vi "Lab Panel V4.88.vi"() -> ()   [LabVIEW 2013] (continued)
                            n2188 = Build Array(w4041) -> (w4037:dbl[])
                            n2189 = Build Array(w4039) -> (w4036:dbl[])
                            n2190 = Build Array(w4044) -> (w4031:dbl[])
                            n2191 = Build Array("AMPS ON", "AMPS OFF", "VOLTS", "PF", "TEMP Live", "TEMP Neut", "CYCLE") -> (w4014:string[])
                            n2192 = Bundle By Name("Y"=w4037, "t0"=w4030) -> (w4029:waveform(dbl))  [unwired: 1 in]
                            n2193 = Bundle By Name("Y"=w4036, "t0"=w4030) -> (w4028:waveform(dbl))  [unwired: 1 in]
                            n2194 = Bundle By Name("Y"=w4035, "t0"=w4030) -> (w4027:waveform(dbl))  [unwired: 1 in]
                            n2195 = Bundle By Name("Y"=w4034, "t0"=w4030) -> (w4026:waveform(dbl))  [unwired: 1 in]
                            n2196 = Bundle By Name("Y"=w4033, "t0"=w4030) -> (w4025:waveform(dbl))  [unwired: 1 in]
                            n2197 = Bundle By Name("Y"=w4032, "t0"=w4030) -> (w4024:waveform(dbl))  [unwired: 1 in]
                            n2198 = Bundle By Name("Y"=w4031, "t0"=w4030) -> (w4023:waveform(dbl))  [unwired: 1 in]
                            n2199 = Build Array(w4029, w4028, w4027, w4026, w4025, w4024, w4023) -> (w4022:waveform(dbl)[])
                            n2200 = TDMS Write(0:w4043, 5:"TEST VALUES", 7:w4014, 9:w4022) -> (4:w4013:refnum<k34>, 6:w4012:string, 15:w4011:errorcluster)  [unwired: 2 in, 1 out]
                            n2201 = TDMS Write(0:w4013, 5:w4012, 7:"TIME", 9:w4009, 11:w4011) -> (15:w4008:errorcluster)  [unwired: 1 in, 3 out]
                            n2202 = local write "data file error"(w4008) -> ()
                          }
                        }
                      }
                    }
                  }
                }
              }
              frame #4 {
                n2203 = case shown="True" w4047 {
                  tunnel: w4051 -> [_ w4056]
                  tunnel: w4050 -> [_ w4055]
                  tunnel: w4049 -> [_ w4053]
                  tunnel: w4048 -> [_ w4052]
                  frame False {
                  }
                  frame True {
                    n2204 = local read "DISP LAB03-1"() -> (w4057:T4)
                    n2205 = local read "SIG LAB03-1"() -> (w4058:T2)
                    n2206 = local read "ON L03-1"() -> (w4054:cluster{"amps":dbl, "volts":dbl, "pf":dbl})
                    n2207 = Unbundle(w4058) -> ("AMPS"=w4064:dbl, "VOLTS"=w4062:dbl, "PF"=w4061:dbl, "Tmp Live"=w4060:dbl, "Tmp Neut"=w4063:dbl)
                    n2208 = Unbundle(w4057) -> ("CYCLE"=w4059:dbl)  [unwired: 2 out]
                    n2209 = stacked-sequence {
                      tunnel: w4064 -> [w4068 w4087]
                      tunnel: w4063 -> [_ w4086]
                      tunnel: w4062 -> [w4067 w4085]
                      tunnel: w4061 -> [w4066 w4084]
                      tunnel: w4060 -> [_ w4083]
                      tunnel: w4059 -> [_ w4082]
                      tunnel: w4056 -> [_ w4081]
                      tunnel: w4055 -> [w4069 _]
                      tunnel: w4054 -> [w4065 w4079]
                      tunnel: w4053 -> [_ w4080]
                      tunnel: w4052 -> [_ w4075]
                      frame #0 {
                        n2210 = case shown="True" w4069 {
                          tunnel: w4068 -> [_ w4074]
                          tunnel: w4067 -> [_ w4073]
                          tunnel: w4066 -> [_ w4072]
                          tunnel: w4065 -> [_ w4070]
                          frame False {
                          }
                          frame True {
                            n2211 = Bundle(cluster=w4070, "amps"=w4074, "volts"=w4073, "pf"=w4072) -> (w4071:cluster{"amps":dbl, "volts":dbl, "pf":dbl})
                            n2212 = local write "ON L03-1"(w4071) -> ()
                          }
                        }
                      }
                      frame #1 {
                        n2213 = Unbundle(w4079) -> ("amps"=w4078:dbl, "volts"=w4077:dbl, "pf"=w4076:dbl)
                        n2214 = case shown="True" w4080 {
                          tunnel: w4087 -> [_ w4119]
                          tunnel: w4086 -> [_ w4126]
                          tunnel: w4085 -> [_ _]
                          tunnel: w4084 -> [_ _]
                          tunnel: w4083 -> [_ w4125]
                          tunnel: w4082 -> [_ w4124]
                          tunnel: w4081 -> [_ w4089]
                          tunnel: w4078 -> [_ w4121]
                          tunnel: w4077 -> [_ w4120]
                          tunnel: w4076 -> [_ w4118]
                          tunnel: w4075 -> [_ w4110]
                          frame False {
                          }
                          frame True {
                            n2215 = local read "TDMS LAB03-1"() -> (w4123:refnum<k34>)
                            n2216 = Build Array(w4120) -> (w4115:dbl[])
                            n2217 = Build Array(w4118) -> (w4114:dbl[])
                            n2218 = Build Array(w4125) -> (w4113:dbl[])
                            n2219 = Build Array(w4126) -> (w4112:dbl[])
                            n2220 = Build Array(w4121) -> (w4117:dbl[])
                            n2221 = Build Array(w4119) -> (w4116:dbl[])
                            n2222 = Build Array(w4124) -> (w4111:dbl[])
                            n2223 = Build Array("AMPS ON", "AMPS OFF", "VOLTS", "PF", "TEMP Live", "TEMP Neut", "CYCLE") -> (w4094:string[])
                            n2224 = Bundle By Name("Y"=w4117, "t0"=w4110) -> (w4109:waveform(dbl))  [unwired: 1 in]
                            n2225 = Bundle By Name("Y"=w4116, "t0"=w4110) -> (w4108:waveform(dbl))  [unwired: 1 in]
                            n2226 = Bundle By Name("Y"=w4115, "t0"=w4110) -> (w4107:waveform(dbl))  [unwired: 1 in]
                            n2227 = Bundle By Name("Y"=w4114, "t0"=w4110) -> (w4106:waveform(dbl))  [unwired: 1 in]
                            n2228 = Bundle By Name("Y"=w4113, "t0"=w4110) -> (w4105:waveform(dbl))  [unwired: 1 in]
                            n2229 = Bundle By Name("Y"=w4112, "t0"=w4110) -> (w4104:waveform(dbl))  [unwired: 1 in]
                            n2230 = Bundle By Name("Y"=w4111, "t0"=w4110) -> (w4103:waveform(dbl))  [unwired: 1 in]
                            n2231 = Build Array(w4109, w4108, w4107, w4106, w4105, w4104, w4103) -> (w4102:waveform(dbl)[])
                            n2232 = TDMS Write(0:w4123, 5:"TEST VALUES", 7:w4094, 9:w4102) -> (4:w4093:refnum<k34>, 6:w4092:string, 15:w4091:errorcluster)  [unwired: 2 in, 1 out]
                            n2233 = TDMS Write(0:w4093, 5:w4092, 7:"TIME", 9:w4089, 11:w4091) -> (15:w4088:errorcluster)  [unwired: 1 in, 3 out]
                            n2234 = local write "data file error"(w4088) -> ()
                          }
                        }
                      }
                    }
                  }
                }
              }
              frame #5 {
                n2235 = case shown="True" w4127 {
                  tunnel: w4131 -> [_ w4136]
                  tunnel: w4130 -> [_ w4135]
                  tunnel: w4129 -> [_ w4133]
                  tunnel: w4128 -> [_ w4132]
                  frame False {
                  }
                  frame True {
                    n2236 = local read "DISP LAB03-2"() -> (w4137:T4)
                    n2237 = local read "SIG LAB03-2"() -> (w4138:T2)
                    n2238 = local read "ON L03-2"() -> (w4134:cluster{"amps":dbl, "volts":dbl, "pf":dbl})
                    n2239 = Unbundle(w4138) -> ("AMPS"=w4144:dbl, "VOLTS"=w4142:dbl, "PF"=w4141:dbl, "Tmp Live"=w4140:dbl, "Tmp Neut"=w4143:dbl)
                    n2240 = Unbundle(w4137) -> ("CYCLE"=w4139:dbl)  [unwired: 2 out]
                    n2241 = stacked-sequence {
                      tunnel: w4144 -> [w4148 w4167]
                      tunnel: w4143 -> [_ w4166]
                      tunnel: w4142 -> [w4147 w4165]
                      tunnel: w4141 -> [w4146 w4164]
                      tunnel: w4140 -> [_ w4163]
                      tunnel: w4139 -> [_ w4162]
                      tunnel: w4136 -> [_ w4161]
                      tunnel: w4135 -> [w4149 _]
                      tunnel: w4134 -> [w4145 w4159]
                      tunnel: w4133 -> [_ w4160]
                      tunnel: w4132 -> [_ w4155]
                      frame #0 {
                        n2242 = case shown="True" w4149 {
                          tunnel: w4148 -> [_ w4154]
                          tunnel: w4147 -> [_ w4153]
                          tunnel: w4146 -> [_ w4152]
                          tunnel: w4145 -> [_ w4150]
                          frame False {
                          }
                          frame True {
                            n2243 = Bundle(cluster=w4150, "amps"=w4154, "volts"=w4153, "pf"=w4152) -> (w4151:cluster{"amps":dbl, "volts":dbl, "pf":dbl})
                            n2244 = local write "ON L03-2"(w4151) -> ()
                          }
                        }
                      }
                      frame #1 {
                        n2245 = Unbundle(w4159) -> ("amps"=w4158:dbl, "volts"=w4157:dbl, "pf"=w4156:dbl)
                        n2246 = case shown="True" w4160 {
                          tunnel: w4167 -> [_ w4199]
                          tunnel: w4166 -> [_ w4206]
                          tunnel: w4165 -> [_ _]
                          tunnel: w4164 -> [_ _]
                          tunnel: w4163 -> [_ w4205]
                          tunnel: w4162 -> [_ w4204]
                          tunnel: w4161 -> [_ w4169]
                          tunnel: w4158 -> [_ w4201]
                          tunnel: w4157 -> [_ w4200]
                          tunnel: w4156 -> [_ w4198]
                          tunnel: w4155 -> [_ w4190]
                          frame False {
                          }
                          frame True {
                            n2247 = local read "TDMS LAB03-2"() -> (w4203:refnum<k34>)
                            n2248 = Build Array(w4200) -> (w4195:dbl[])
                            n2249 = Build Array(w4198) -> (w4194:dbl[])
                            n2250 = Build Array(w4205) -> (w4193:dbl[])
                            n2251 = Build Array(w4206) -> (w4192:dbl[])
                            n2252 = Build Array(w4201) -> (w4197:dbl[])
                            n2253 = Build Array(w4199) -> (w4196:dbl[])
                            n2254 = Build Array(w4204) -> (w4191:dbl[])
                            n2255 = Build Array("AMPS ON", "AMPS OFF", "VOLTS", "PF", "TEMP Live", "TEMP Neut", "CYCLE") -> (w4174:string[])
                            n2256 = Bundle By Name("Y"=w4197, "t0"=w4190) -> (w4189:waveform(dbl))  [unwired: 1 in]
                            n2257 = Bundle By Name("Y"=w4196, "t0"=w4190) -> (w4188:waveform(dbl))  [unwired: 1 in]
                            n2258 = Bundle By Name("Y"=w4195, "t0"=w4190) -> (w4187:waveform(dbl))  [unwired: 1 in]
                            n2259 = Bundle By Name("Y"=w4194, "t0"=w4190) -> (w4186:waveform(dbl))  [unwired: 1 in]
                            n2260 = Bundle By Name("Y"=w4193, "t0"=w4190) -> (w4185:waveform(dbl))  [unwired: 1 in]
                            n2261 = Bundle By Name("Y"=w4192, "t0"=w4190) -> (w4184:waveform(dbl))  [unwired: 1 in]
                            n2262 = Bundle By Name("Y"=w4191, "t0"=w4190) -> (w4183:waveform(dbl))  [unwired: 1 in]
                            n2263 = Build Array(w4189, w4188, w4187, w4186, w4185, w4184, w4183) -> (w4182:waveform(dbl)[])
                            n2264 = TDMS Write(0:w4203, 5:"TEST VALUES", 7:w4174, 9:w4182) -> (4:w4173:refnum<k34>, 6:w4172:string, 15:w4171:errorcluster)  [unwired: 2 in, 1 out]
                            n2265 = TDMS Write(0:w4173, 5:w4172, 7:"TIME", 9:w4169, 11:w4171) -> (15:w4168:errorcluster)  [unwired: 1 in, 3 out]
                            n2266 = local write "data file error"(w4168) -> ()
                          }
                        }
                      }
                    }
                  }
                }
              }
              frame #6 {
                n2267 = case shown="True" w4207 {
                  tunnel: w4211 -> [_ w4216]
                  tunnel: w4210 -> [_ w4215]
                  tunnel: w4209 -> [_ w4213]
                  tunnel: w4208 -> [_ w4212]
                  frame False {
                  }
                  frame True {
                    n2268 = local read "DISP LAB04-1"() -> (w4217:T4)
                    n2269 = local read "SIG LAB04-1"() -> (w4218:T2)
                    n2270 = local read "ON L04-1"() -> (w4214:cluster{"amps":dbl, "volts":dbl, "pf":dbl})
                    n2271 = Unbundle(w4218) -> ("AMPS"=w4224:dbl, "VOLTS"=w4222:dbl, "PF"=w4221:dbl, "Tmp Live"=w4220:dbl, "Tmp Neut"=w4223:dbl)
                    n2272 = Unbundle(w4217) -> ("CYCLE"=w4219:dbl)  [unwired: 2 out]
                    n2273 = stacked-sequence {
                      tunnel: w4224 -> [w4228 w4247]
                      tunnel: w4223 -> [_ w4246]
                      tunnel: w4222 -> [w4227 w4245]
                      tunnel: w4221 -> [w4226 w4244]
                      tunnel: w4220 -> [_ w4243]
                      tunnel: w4219 -> [_ w4242]
                      tunnel: w4216 -> [_ w4241]
                      tunnel: w4215 -> [w4229 _]
                      tunnel: w4214 -> [w4225 w4239]
                      tunnel: w4213 -> [_ w4240]
                      tunnel: w4212 -> [_ w4235]
                      frame #0 {
                        n2274 = case shown="True" w4229 {
                          tunnel: w4228 -> [_ w4234]
                          tunnel: w4227 -> [_ w4233]
                          tunnel: w4226 -> [_ w4232]
                          tunnel: w4225 -> [_ w4230]
                          frame False {
                          }
                          frame True {
                            n2275 = Bundle(cluster=w4230, "amps"=w4234, "volts"=w4233, "pf"=w4232) -> (w4231:cluster{"amps":dbl, "volts":dbl, "pf":dbl})
                            n2276 = local write "ON L04-1"(w4231) -> ()
                          }
                        }
                      }
                      frame #1 {
                        n2277 = Unbundle(w4239) -> ("amps"=w4238:dbl, "volts"=w4237:dbl, "pf"=w4236:dbl)
                        n2278 = case shown="True" w4240 {
                          tunnel: w4247 -> [_ w4279]
                          tunnel: w4246 -> [_ w4286]
                          tunnel: w4245 -> [_ _]
                          tunnel: w4244 -> [_ _]
                          tunnel: w4243 -> [_ w4285]
                          tunnel: w4242 -> [_ w4284]
                          tunnel: w4241 -> [_ w4249]
                          tunnel: w4238 -> [_ w4281]
                          tunnel: w4237 -> [_ w4280]
                          tunnel: w4236 -> [_ w4278]
                          tunnel: w4235 -> [_ w4270]
                          frame False {
                          }
                          frame True {
                            n2279 = local read "TDMS LAB04-1"() -> (w4283:refnum<k34>)
                            n2280 = Build Array(w4280) -> (w4275:dbl[])
                            n2281 = Build Array(w4278) -> (w4274:dbl[])
                            n2282 = Build Array(w4285) -> (w4273:dbl[])
                            n2283 = Build Array(w4286) -> (w4272:dbl[])
                            n2284 = Build Array(w4281) -> (w4277:dbl[])
                            n2285 = Build Array(w4279) -> (w4276:dbl[])
                            n2286 = Build Array(w4284) -> (w4271:dbl[])
                            n2287 = Build Array("AMPS ON", "AMPS OFF", "VOLTS", "PF", "TEMP Live", "TEMP Neut", "CYCLE") -> (w4254:string[])
                            n2288 = Bundle By Name("Y"=w4277, "t0"=w4270) -> (w4269:waveform(dbl))  [unwired: 1 in]
                            n2289 = Bundle By Name("Y"=w4276, "t0"=w4270) -> (w4268:waveform(dbl))  [unwired: 1 in]
                            n2290 = Bundle By Name("Y"=w4275, "t0"=w4270) -> (w4267:waveform(dbl))  [unwired: 1 in]
                            n2291 = Bundle By Name("Y"=w4274, "t0"=w4270) -> (w4266:waveform(dbl))  [unwired: 1 in]
                            n2292 = Bundle By Name("Y"=w4273, "t0"=w4270) -> (w4265:waveform(dbl))  [unwired: 1 in]
                            n2293 = Bundle By Name("Y"=w4272, "t0"=w4270) -> (w4264:waveform(dbl))  [unwired: 1 in]
                            n2294 = Bundle By Name("Y"=w4271, "t0"=w4270) -> (w4263:waveform(dbl))  [unwired: 1 in]
                            n2295 = Build Array(w4269, w4268, w4267, w4266, w4265, w4264, w4263) -> (w4262:waveform(dbl)[])
                            n2296 = TDMS Write(0:w4283, 5:"TEST VALUES", 7:w4254, 9:w4262) -> (4:w4253:refnum<k34>, 6:w4252:string, 15:w4251:errorcluster)  [unwired: 2 in, 1 out]
                            n2297 = TDMS Write(0:w4253, 5:w4252, 7:"TIME", 9:w4249, 11:w4251) -> (15:w4248:errorcluster)  [unwired: 1 in, 3 out]
                            n2298 = local write "data file error"(w4248) -> ()
                          }
                        }
                      }
                    }
                  }
                }
              }
              frame #7 {
                n2299 = case shown="True" w4287 {
                  tunnel: w4291 -> [_ w4296]
                  tunnel: w4290 -> [_ w4295]
                  tunnel: w4289 -> [_ w4293]
                  tunnel: w4288 -> [_ w4292]
                  frame False {
                  }
                  frame True {
                    n2300 = local read "DISP LAB04-2"() -> (w4297:T4)
                    n2301 = local read "SIG LAB04-2"() -> (w4298:T2)
                    n2302 = local read "ON L04-2"() -> (w4294:cluster{"amps":dbl, "volts":dbl, "pf":dbl})
                    n2303 = Unbundle(w4298) -> ("AMPS"=w4304:dbl, "VOLTS"=w4302:dbl, "PF"=w4301:dbl, "Tmp Live"=w4300:dbl, "Tmp Neut"=w4303:dbl)
                    n2304 = Unbundle(w4297) -> ("CYCLE"=w4299:dbl)  [unwired: 2 out]
                    n2305 = stacked-sequence {
                      tunnel: w4304 -> [w4308 w4327]
                      tunnel: w4303 -> [_ w4326]
                      tunnel: w4302 -> [w4307 w4325]
                      tunnel: w4301 -> [w4306 w4324]
                      tunnel: w4300 -> [_ w4323]
                      tunnel: w4299 -> [_ w4322]
                      tunnel: w4296 -> [_ w4321]
                      tunnel: w4295 -> [w4309 _]
                      tunnel: w4294 -> [w4305 w4319]
                      tunnel: w4293 -> [_ w4320]
                      tunnel: w4292 -> [_ w4315]
                      frame #0 {
                        n2306 = case shown="True" w4309 {
                          tunnel: w4308 -> [_ w4314]
                          tunnel: w4307 -> [_ w4313]
                          tunnel: w4306 -> [_ w4312]
                          tunnel: w4305 -> [_ w4310]
                          frame False {
                          }
                          frame True {
                            n2307 = Bundle(cluster=w4310, "amps"=w4314, "volts"=w4313, "pf"=w4312) -> (w4311:cluster{"amps":dbl, "volts":dbl, "pf":dbl})
                            n2308 = local write "ON L04-2"(w4311) -> ()
                          }
                        }
                      }
                      frame #1 {
                        n2309 = Unbundle(w4319) -> ("amps"=w4318:dbl, "volts"=w4317:dbl, "pf"=w4316:dbl)
                        n2310 = case shown="True" w4320 {
                          tunnel: w4327 -> [_ w4359]
                          tunnel: w4326 -> [_ w4366]
                          tunnel: w4325 -> [_ _]
                          tunnel: w4324 -> [_ _]
                          tunnel: w4323 -> [_ w4365]
                          tunnel: w4322 -> [_ w4364]
                          tunnel: w4321 -> [_ w4329]
                          tunnel: w4318 -> [_ w4361]
                          tunnel: w4317 -> [_ w4360]
                          tunnel: w4316 -> [_ w4358]
                          tunnel: w4315 -> [_ w4350]
                          frame False {
                          }
                          frame True {
                            n2311 = local read "TDMS LAB04-2"() -> (w4363:refnum<k34>)
                            n2312 = Build Array(w4360) -> (w4355:dbl[])
                            n2313 = Build Array(w4358) -> (w4354:dbl[])
                            n2314 = Build Array(w4365) -> (w4353:dbl[])
                            n2315 = Build Array(w4366) -> (w4352:dbl[])
                            n2316 = Build Array(w4361) -> (w4357:dbl[])
                            n2317 = Build Array(w4359) -> (w4356:dbl[])
                            n2318 = Build Array(w4364) -> (w4351:dbl[])
                            n2319 = Build Array("AMPS ON", "AMPS OFF", "VOLTS", "PF", "TEMP Live", "TEMP Neut", "CYCLE") -> (w4334:string[])
                            n2320 = Bundle By Name("Y"=w4357, "t0"=w4350) -> (w4349:waveform(dbl))  [unwired: 1 in]
                            n2321 = Bundle By Name("Y"=w4356, "t0"=w4350) -> (w4348:waveform(dbl))  [unwired: 1 in]
                            n2322 = Bundle By Name("Y"=w4355, "t0"=w4350) -> (w4347:waveform(dbl))  [unwired: 1 in]
                            n2323 = Bundle By Name("Y"=w4354, "t0"=w4350) -> (w4346:waveform(dbl))  [unwired: 1 in]
                            n2324 = Bundle By Name("Y"=w4353, "t0"=w4350) -> (w4345:waveform(dbl))  [unwired: 1 in]
                            n2325 = Bundle By Name("Y"=w4352, "t0"=w4350) -> (w4344:waveform(dbl))  [unwired: 1 in]
                            n2326 = Bundle By Name("Y"=w4351, "t0"=w4350) -> (w4343:waveform(dbl))  [unwired: 1 in]
                            n2327 = Build Array(w4349, w4348, w4347, w4346, w4345, w4344, w4343) -> (w4342:waveform(dbl)[])
                            n2328 = TDMS Write(0:w4363, 5:"TEST VALUES", 7:w4334, 9:w4342) -> (4:w4333:refnum<k34>, 6:w4332:string, 15:w4331:errorcluster)  [unwired: 2 in, 1 out]
                            n2329 = TDMS Write(0:w4333, 5:w4332, 7:"TIME", 9:w4329, 11:w4331) -> (15:w4328:errorcluster)  [unwired: 1 in, 3 out]
                            n2330 = local write "data file error"(w4328) -> ()
                          }
                        }
                      }
                    }
                  }
                }
              }
              frame #8 {
                n2331 = case shown="True" w4367 {
                  tunnel: w4371 -> [_ w4376]
                  tunnel: w4370 -> [_ w4375]
                  tunnel: w4369 -> [_ w4373]
                  tunnel: w4368 -> [_ w4372]
                  frame False {
                  }
                  frame True {
                    n2332 = local read "DISP LAB05-1"() -> (w4377:T4)
                    n2333 = local read "SIG LAB05-1"() -> (w4378:T2)
                    n2334 = local read "ON L05-1"() -> (w4374:cluster{"amps":dbl, "volts":dbl, "pf":dbl})
                    n2335 = Unbundle(w4378) -> ("AMPS"=w4384:dbl, "VOLTS"=w4382:dbl, "PF"=w4381:dbl, "Tmp Live"=w4380:dbl, "Tmp Neut"=w4383:dbl)
                    n2336 = Unbundle(w4377) -> ("CYCLE"=w4379:dbl)  [unwired: 2 out]
                    n2337 = stacked-sequence {
                      tunnel: w4384 -> [w4388 w4407]
                      tunnel: w4383 -> [_ w4406]
                      tunnel: w4382 -> [w4387 w4405]
                      tunnel: w4381 -> [w4386 w4404]
                      tunnel: w4380 -> [_ w4403]
                      tunnel: w4379 -> [_ w4402]
                      tunnel: w4376 -> [_ w4401]
                      tunnel: w4375 -> [w4389 _]
                      tunnel: w4374 -> [w4385 w4399]
                      tunnel: w4373 -> [_ w4400]
                      tunnel: w4372 -> [_ w4395]
                      frame #0 {
                        n2338 = case shown="True" w4389 {
                          tunnel: w4388 -> [_ w4394]
                          tunnel: w4387 -> [_ w4393]
                          tunnel: w4386 -> [_ w4392]
                          tunnel: w4385 -> [_ w4390]
                          frame False {
                          }
                          frame True {
                            n2339 = Bundle(cluster=w4390, "amps"=w4394, "volts"=w4393, "pf"=w4392) -> (w4391:cluster{"amps":dbl, "volts":dbl, "pf":dbl})
                            n2340 = local write "ON L05-1"(w4391) -> ()
                          }
                        }
                      }
                      frame #1 {
                        n2341 = Unbundle(w4399) -> ("amps"=w4398:dbl, "volts"=w4397:dbl, "pf"=w4396:dbl)
                        n2342 = case shown="True" w4400 {
                          tunnel: w4407 -> [_ w4439]
                          tunnel: w4406 -> [_ w4446]
                          tunnel: w4405 -> [_ _]
                          tunnel: w4404 -> [_ _]
                          tunnel: w4403 -> [_ w4445]
                          tunnel: w4402 -> [_ w4444]
                          tunnel: w4401 -> [_ w4409]
                          tunnel: w4398 -> [_ w4441]
                          tunnel: w4397 -> [_ w4440]
                          tunnel: w4396 -> [_ w4438]
                          tunnel: w4395 -> [_ w4430]
                          frame False {
                          }
                          frame True {
                            n2343 = local read "TDMS LAB05-1"() -> (w4443:refnum<k34>)
                            n2344 = Build Array(w4440) -> (w4435:dbl[])
                            n2345 = Build Array(w4438) -> (w4434:dbl[])
                            n2346 = Build Array(w4445) -> (w4433:dbl[])
                            n2347 = Build Array(w4446) -> (w4432:dbl[])
                            n2348 = Build Array(w4441) -> (w4437:dbl[])
                            n2349 = Build Array(w4439) -> (w4436:dbl[])
                            n2350 = Build Array(w4444) -> (w4431:dbl[])
                            n2351 = Build Array("AMPS ON", "AMPS OFF", "VOLTS", "PF", "TEMP Live", "TEMP Neut", "CYCLE") -> (w4414:string[])
                            n2352 = Bundle By Name("Y"=w4437, "t0"=w4430) -> (w4429:waveform(dbl))  [unwired: 1 in]
                            n2353 = Bundle By Name("Y"=w4436, "t0"=w4430) -> (w4428:waveform(dbl))  [unwired: 1 in]
                            n2354 = Bundle By Name("Y"=w4435, "t0"=w4430) -> (w4427:waveform(dbl))  [unwired: 1 in]
                            n2355 = Bundle By Name("Y"=w4434, "t0"=w4430) -> (w4426:waveform(dbl))  [unwired: 1 in]
                            n2356 = Bundle By Name("Y"=w4433, "t0"=w4430) -> (w4425:waveform(dbl))  [unwired: 1 in]
                            n2357 = Bundle By Name("Y"=w4432, "t0"=w4430) -> (w4424:waveform(dbl))  [unwired: 1 in]
                            n2358 = Bundle By Name("Y"=w4431, "t0"=w4430) -> (w4423:waveform(dbl))  [unwired: 1 in]
                            n2359 = Build Array(w4429, w4428, w4427, w4426, w4425, w4424, w4423) -> (w4422:waveform(dbl)[])
                            n2360 = TDMS Write(0:w4443, 5:"TEST VALUES", 7:w4414, 9:w4422) -> (4:w4413:refnum<k34>, 6:w4412:string, 15:w4411:errorcluster)  [unwired: 2 in, 1 out]
                            n2361 = TDMS Write(0:w4413, 5:w4412, 7:"TIME", 9:w4409, 11:w4411) -> (15:w4408:errorcluster)  [unwired: 1 in, 3 out]
                            n2362 = local write "data file error"(w4408) -> ()
                          }
                        }
                      }
                    }
                  }
                }
              }
              frame #9 {
                n2363 = case shown="True" w4447 {
                  tunnel: w4451 -> [_ w4456]
                  tunnel: w4450 -> [_ w4455]
                  tunnel: w4449 -> [_ w4453]
                  tunnel: w4448 -> [_ w4452]
                  frame False {
                  }
                  frame True {
                    n2364 = local read "DISP LAB05-2"() -> (w4457:T4)
                    n2365 = local read "SIG LAB05-2"() -> (w4458:T2)
                    n2366 = local read "ON L05-2"() -> (w4454:cluster{"amps":dbl, "volts":dbl, "pf":dbl})
                    n2367 = Unbundle(w4458) -> ("AMPS"=w4464:dbl, "VOLTS"=w4462:dbl, "PF"=w4461:dbl, "Tmp Live"=w4460:dbl, "Tmp Neut"=w4463:dbl)
                    n2368 = Unbundle(w4457) -> ("CYCLE"=w4459:dbl)  [unwired: 2 out]
                    n2369 = stacked-sequence {
                      tunnel: w4464 -> [w4468 w4487]
                      tunnel: w4463 -> [_ w4486]
                      tunnel: w4462 -> [w4467 w4485]
                      tunnel: w4461 -> [w4466 w4484]
                      tunnel: w4460 -> [_ w4483]
                      tunnel: w4459 -> [_ w4482]
                      tunnel: w4456 -> [_ w4481]
                      tunnel: w4455 -> [w4469 _]
                      tunnel: w4454 -> [w4465 w4479]
                      tunnel: w4453 -> [_ w4480]
                      tunnel: w4452 -> [_ w4475]
                      frame #0 {
                        n2370 = case shown="True" w4469 {
                          tunnel: w4468 -> [_ w4474]
                          tunnel: w4467 -> [_ w4473]
                          tunnel: w4466 -> [_ w4472]
                          tunnel: w4465 -> [_ w4470]
                          frame False {
                          }
                          frame True {
                            n2371 = Bundle(cluster=w4470, "amps"=w4474, "volts"=w4473, "pf"=w4472) -> (w4471:cluster{"amps":dbl, "volts":dbl, "pf":dbl})
                            n2372 = local write "ON L05-2"(w4471) -> ()
                          }
                        }
                      }
                      frame #1 {
                        n2373 = Unbundle(w4479) -> ("amps"=w4478:dbl, "volts"=w4477:dbl, "pf"=w4476:dbl)
                        n2374 = case shown="True" w4480 {
                          tunnel: w4487 -> [_ w4519]
                          tunnel: w4486 -> [_ w4526]
                          tunnel: w4485 -> [_ _]
                          tunnel: w4484 -> [_ _]
                          tunnel: w4483 -> [_ w4525]
                          tunnel: w4482 -> [_ w4524]
                          tunnel: w4481 -> [_ w4489]
                          tunnel: w4478 -> [_ w4521]
                          tunnel: w4477 -> [_ w4520]
                          tunnel: w4476 -> [_ w4518]
                          tunnel: w4475 -> [_ w4510]
                          frame False {
                          }
                          frame True {
                            n2375 = local read "TDMS LAB05-2"() -> (w4523:refnum<k34>)
                            n2376 = Build Array(w4520) -> (w4515:dbl[])
                            n2377 = Build Array(w4518) -> (w4514:dbl[])
                            n2378 = Build Array(w4525) -> (w4513:dbl[])
                            n2379 = Build Array(w4526) -> (w4512:dbl[])
                            n2380 = Build Array(w4521) -> (w4517:dbl[])
                            n2381 = Build Array(w4519) -> (w4516:dbl[])
                            n2382 = Build Array(w4524) -> (w4511:dbl[])
                            n2383 = Build Array("AMPS ON", "AMPS OFF", "VOLTS", "PF", "TEMP Live", "TEMP Neut", "CYCLE") -> (w4494:string[])
                            n2384 = Bundle By Name("Y"=w4517, "t0"=w4510) -> (w4509:waveform(dbl))  [unwired: 1 in]
                            n2385 = Bundle By Name("Y"=w4516, "t0"=w4510) -> (w4508:waveform(dbl))  [unwired: 1 in]
                            n2386 = Bundle By Name("Y"=w4515, "t0"=w4510) -> (w4507:waveform(dbl))  [unwired: 1 in]
                            n2387 = Bundle By Name("Y"=w4514, "t0"=w4510) -> (w4506:waveform(dbl))  [unwired: 1 in]
                            n2388 = Bundle By Name("Y"=w4513, "t0"=w4510) -> (w4505:waveform(dbl))  [unwired: 1 in]
                            n2389 = Bundle By Name("Y"=w4512, "t0"=w4510) -> (w4504:waveform(dbl))  [unwired: 1 in]
                            n2390 = Bundle By Name("Y"=w4511, "t0"=w4510) -> (w4503:waveform(dbl))  [unwired: 1 in]
                            n2391 = Build Array(w4509, w4508, w4507, w4506, w4505, w4504, w4503) -> (w4502:waveform(dbl)[])
                            n2392 = TDMS Write(0:w4523, 5:"TEST VALUES", 7:w4494, 9:w4502) -> (4:w4493:refnum<k34>, 6:w4492:string, 15:w4491:errorcluster)  [unwired: 2 in, 1 out]
                            n2393 = TDMS Write(0:w4493, 5:w4492, 7:"TIME", 9:w4489, 11:w4491) -> (15:w4488:errorcluster)  [unwired: 1 in, 3 out]
                            n2394 = local write "data file error"(w4488) -> ()
                          }
                        }
                      }
                    }
                  }
                }
              }
            }
          }
          frame #13 {
            # "display test values on chart"
            n2395 = local read "jig cycle"() -> (w4531:dbl)
            n2396 = local read "on loops"() -> (w4533:dbl)
            n2397 = Add(x=w4533, y=2) -> (x+y=w4530:dbl)
            n2398 = Equal?(x=w4531, y=1) -> (x = y?=w4529:bool)
            n2399 = Equal?(x=w4531, y=w4530) -> (x = y?=w4528:bool)
            n2400 = Or(x=w4529, y=w4528) -> (x .or. y?=w4527:bool)
            "graph flag" <- w4527
            n2401 = global write "Global display 3.vi" "graph flag"(w4527) -> ()
            n2402 = case shown="True" w4527 {
              frame False {
              }
              frame True {
                n2403 = local read "SIG LAB05-1"() -> (w4576:T2)
                n2404 = local read "SIG LAB04-2"() -> (w4577:T2)
                n2405 = local read "SIG LAB05-2"() -> (w4575:T2)
                n2406 = local read "SIG LAB04-1"() -> (w4578:T2)
                n2407 = local read "SIG LAB03-1"() -> (w4580:T2)
                n2408 = local read "SIG LAB03-2"() -> (w4579:T2)
                n2409 = local read "SIG LAB01-1"() -> (w4584:T2)
                n2410 = local read "SIG LAB02-2"() -> (w4581:T2)
                n2411 = local read "SIG LAB02-1"() -> (w4582:T2)
                n2412 = local read "SIG LAB01-2"() -> (w4583:T2)
                n2413 = Unbundle(w4577) -> ("AMPS"=w4567:dbl, "VOLTS"=w4557:dbl, "Tmp Live"=w4547:dbl, "Tmp Neut"=w4537:dbl)  [unwired: 1 out]
                n2414 = Unbundle(w4576) -> ("AMPS"=w4566:dbl, "VOLTS"=w4556:dbl, "Tmp Live"=w4546:dbl, "Tmp Neut"=w4536:dbl)  [unwired: 1 out]
                n2415 = Unbundle(w4575) -> ("AMPS"=w4565:dbl, "VOLTS"=w4555:dbl, "Tmp Live"=w4545:dbl, "Tmp Neut"=w4535:dbl)  [unwired: 1 out]
                n2416 = Unbundle(w4578) -> ("AMPS"=w4568:dbl, "VOLTS"=w4558:dbl, "Tmp Live"=w4548:dbl, "Tmp Neut"=w4538:dbl)  [unwired: 1 out]
                n2417 = Unbundle(w4579) -> ("AMPS"=w4569:dbl, "VOLTS"=w4559:dbl, "Tmp Live"=w4549:dbl, "Tmp Neut"=w4539:dbl)  [unwired: 1 out]
                n2418 = Unbundle(w4580) -> ("AMPS"=w4570:dbl, "VOLTS"=w4560:dbl, "Tmp Live"=w4550:dbl, "Tmp Neut"=w4540:dbl)  [unwired: 1 out]
                n2419 = Unbundle(w4581) -> ("AMPS"=w4571:dbl, "VOLTS"=w4561:dbl, "Tmp Live"=w4551:dbl, "Tmp Neut"=w4541:dbl)  [unwired: 1 out]
                n2420 = Unbundle(w4582) -> ("AMPS"=w4572:dbl, "VOLTS"=w4562:dbl, "Tmp Live"=w4552:dbl, "Tmp Neut"=w4542:dbl)  [unwired: 1 out]
                n2421 = Unbundle(w4584) -> ("AMPS"=w4574:dbl, "VOLTS"=w4564:dbl, "Tmp Live"=w4554:dbl, "Tmp Neut"=w4544:dbl)  [unwired: 1 out]
                n2422 = Unbundle(w4583) -> ("AMPS"=w4573:dbl, "VOLTS"=w4563:dbl, "Tmp Live"=w4553:dbl, "Tmp Neut"=w4543:dbl)  [unwired: 1 out]
                n2423 = stacked-sequence {
                  tunnel: w4574 -> [w4616 _ _]
                  tunnel: w4573 -> [w4615 _ _]
                  tunnel: w4572 -> [w4606 _ _]
                  tunnel: w4571 -> [w4605 _ _]
                  tunnel: w4570 -> [w4595 _ _]
                  tunnel: w4569 -> [w4594 _ _]
                  tunnel: w4568 -> [_ w4639 _]
                  tunnel: w4567 -> [_ w4638 _]
                  tunnel: w4566 -> [_ w4628 _]
                  tunnel: w4565 -> [_ w4627 _]
                  tunnel: w4564 -> [w4613 _ _]
                  tunnel: w4563 -> [w4612 _ _]
                  tunnel: w4562 -> [w4603 _ _]
                  tunnel: w4561 -> [w4602 _ _]
                  tunnel: w4560 -> [w4593 _ _]
                  tunnel: w4559 -> [w4592 _ _]
                  tunnel: w4558 -> [_ w4637 _]
                  tunnel: w4557 -> [_ w4636 _]
                  tunnel: w4556 -> [_ w4626 _]
                  tunnel: w4555 -> [_ w4625 _]
                  tunnel: w4554 -> [w4610 _ _]
                  tunnel: w4553 -> [w4608 _ _]
                  tunnel: w4552 -> [w4599 _ _]
                  tunnel: w4551 -> [w4597 _ _]
                  tunnel: w4550 -> [w4591 _ _]
                  tunnel: w4549 -> [w4589 _ _]
                  tunnel: w4548 -> [_ w4635 _]
                  tunnel: w4547 -> [_ w4633 _]
                  tunnel: w4546 -> [_ w4624 _]
                  tunnel: w4545 -> [_ w4622 _]
                  tunnel: w4544 -> [w4609 _ _]
                  tunnel: w4543 -> [w4607 _ _]
                  tunnel: w4542 -> [w4598 _ _]
                  tunnel: w4541 -> [w4596 _ _]
                  tunnel: w4540 -> [w4590 _ _]
                  tunnel: w4539 -> [w4588 _ _]
                  tunnel: w4538 -> [_ w4634 _]
                  tunnel: w4537 -> [_ w4632 _]
                  tunnel: w4536 -> [_ w4623 _]
                  tunnel: w4535 -> [_ w4621 _]
                  frame #0 {
                    n2424 = Merge Signals(w4616, w4615) -> (→"LAB01 AMPS":dynamicdata)
                    n2425 = Merge Signals(w4613, w4612) -> (→"LAB01 VOLTS":dynamicdata)
                    n2426 = Merge Signals(w4593, w4592) -> (→"LAB03 VOLTS":dynamicdata)
                    n2427 = Merge Signals(w4610, w4609, w4608, w4607) -> (→"LAB01 deg C":dynamicdata)
                    n2428 = Merge Signals(w4606, w4605) -> (→"LAB02 AMPS":dynamicdata)
                    n2429 = Merge Signals(w4599, w4598, w4597, w4596) -> (→"LAB02 deg C":dynamicdata)
                    n2430 = Merge Signals(w4591, w4590, w4589, w4588) -> (→"LAB03 deg C":dynamicdata)
                    n2431 = Merge Signals(w4603, w4602) -> (→"LAB02 VOLTS":dynamicdata)
                    n2432 = Merge Signals(w4595, w4594) -> (→"LAB03 AMPS":dynamicdata)
                  }
                  frame #1 {
                    n2433 = Merge Signals(w4626, w4625) -> (→"LAB05 VOLTS":dynamicdata)
                    n2434 = Merge Signals(w4639, w4638) -> (→"LAB04 AMPS":dynamicdata)
                    n2435 = Merge Signals(w4628, w4627) -> (→"LAB05 AMPS":dynamicdata)
                    n2436 = Merge Signals(w4624, w4623, w4622, w4621) -> (→"LAB05 deg C":dynamicdata)
                    n2437 = Merge Signals(w4635, w4634, w4633, w4632) -> (→"LAB04 deg C":dynamicdata)
                    n2438 = Merge Signals(w4637, w4636) -> (→"LAB04 VOLTS":dynamicdata)
                  }
                  frame #2 {
                    n2439 = local read "LAB05 VOLTS"() -> (w4647:dynamicdata)
                    n2440 = local read "LAB04 VOLTS"() -> (w4648:dynamicdata)
                    n2441 = local read "LAB02 VOLTS"() -> (w4650:dynamicdata)
                    n2442 = local read "LAB03 VOLTS"() -> (w4649:dynamicdata)
                    n2443 = local read "LAB05 AMPS"() -> (w4653:dynamicdata)
                    n2444 = local read "LAB01 VOLTS"() -> (w4651:dynamicdata)
                    n2445 = local read "LAB04 AMPS"() -> (w4654:dynamicdata)
                    n2446 = local read "LAB03 AMPS"() -> (w4655:dynamicdata)
                    n2447 = local read "LAB03 deg C"() -> (w4643:dynamicdata)
                    n2448 = local read "LAB02 AMPS"() -> (w4656:dynamicdata)
                    n2449 = local read "LAB04 deg C"() -> (w4642:dynamicdata)
                    n2450 = local read "LAB05 deg C"() -> (w4641:dynamicdata)
                    n2451 = local read "LAB02 deg C"() -> (w4644:dynamicdata)
                    n2452 = local read "LAB01 deg C"() -> (w4645:dynamicdata)
                    n2453 = local read "LAB01 AMPS"() -> (w4657:dynamicdata)
                    n2454 = Merge Signals(w4645, w4644, w4643, w4642, w4641) -> (w4640:dynamicdata)
                    n2455 = Merge Signals(w4657, w4656, w4655, w4654, w4653) -> (w4652:dynamicdata)
                    n2456 = Merge Signals(w4651, w4650, w4649, w4648, w4647) -> (w4646:dynamicdata)
                    n2457 = global write "Global display 3.vi" "graph volts"(w4646) -> ()
                    n2458 = global write "Global display 3.vi" "graph deg C"(w4640) -> ()
                    n2459 = global write "Global display 3.vi" "graph amps"(w4652) -> ()
                  }
                }
              }
            }
          }
          frame #14 {
            # "check for amps fail"
            # "check for cycle test & temperature rise fail conditions"
            n2460 = local read "on loops"() -> (w4684:dbl)
            n2461 = local read "jig cycle"() -> (w4681:dbl)
            n2462 = local read "jig cycle"() -> (w4686:dbl)
            n2463 = Add(x=w4684, y=3.0) -> (x+y=w4682:dbl)
            n2464 = Equal?(x=w4681, y=w4682) -> (x = y?=w4677:bool)
            n2465 = local read "Fail Loops"() -> (w4658:dbl)
            n2466 = Equal?(x=w4686, y=1.0) -> (x = y?=w4679:bool)
            n2467 = global write "Global 1.vi" "fail count"(w4658) -> ()
            n2468 = stacked-sequence {
              tunnel: w4680 -> [w4689 _ _ _ _ _ _ _ _ _]
              tunnel: w4679 -> [w4690 w4710 w4730 w4750 w4770 w4790 w4810 w4830 w4850 w4870]
              tunnel: w4678 -> [w4687 _ _ _ _ _ _ _ _ _]
              tunnel: w4677 -> [w4688 w4709 w4729 w4749 w4769 w4789 w4809 w4829 w4849 w4869]
              tunnel: w4676 -> [_ w4708 _ _ _ _ _ _ _ _]
              tunnel: w4675 -> [_ w4707 _ _ _ _ _ _ _ _]
              tunnel: w4674 -> [_ _ w4728 _ _ _ _ _ _ _]
              tunnel: w4673 -> [_ _ w4727 _ _ _ _ _ _ _]
              tunnel: w4672 -> [_ _ _ w4748 _ _ _ _ _ _]
              tunnel: w4671 -> [_ _ _ w4747 _ _ _ _ _ _]
              tunnel: w4670 -> [_ _ _ _ w4768 _ _ _ _ _]
              tunnel: w4669 -> [_ _ _ _ w4767 _ _ _ _ _]
              tunnel: w4668 -> [_ _ _ _ _ w4788 _ _ _ _]
              tunnel: w4667 -> [_ _ _ _ _ w4787 _ _ _ _]
              tunnel: w4666 -> [_ _ _ _ _ _ w4808 _ _ _]
              tunnel: w4665 -> [_ _ _ _ _ _ w4807 _ _ _]
              tunnel: w4664 -> [_ _ _ _ _ _ _ w4828 _ _]
              tunnel: w4663 -> [_ _ _ _ _ _ _ w4827 _ _]
              tunnel: w4662 -> [_ _ _ _ _ _ _ _ w4848 _]
              tunnel: w4661 -> [_ _ _ _ _ _ _ _ w4847 _]
              tunnel: w4660 -> [_ _ _ _ _ _ _ _ _ w4868]
              tunnel: w4659 -> [_ _ _ _ _ _ _ _ _ w4867]
              frame #0 {
                # "LAB01-1"
                n2469 = case shown="True" w4687 {
                  tunnel: w4690 -> [_ w4703]
                  tunnel: w4689 -> [_ w4700]
                  tunnel: w4688 -> [_ w4699]
                  frame False {
                  }
                  frame True {
                    n2470 = local read "TEMP START LAB01-1"() -> (w4705:cluster{"TL":dbl, "TN":dbl})
                    n2471 = local read "RESULT LAB01-1"() -> (w4694:bool)
                    n2472 = local read "FAIL LAB01-1"() -> (w4697:cluster{"LO":dbl, "HI":dbl})
                    n2473 = local read "TDMS LAB01-1"() -> (w4704:refnum<k34>)
                    n2474 = local read "SET LAB01-1"() -> (w4701:T5)
                    n2475 = local read "DISP LAB01-1"() -> (w4702:T4)
                    n2476 = local read "SIG LAB01-1"() -> (w4706:T2)
                    n2477 = Bundle("FAIL LAB01-1"=w4697, "SIG LAB01-1"=w4706, "TEMP START LAB01-1"=w4705, "DISP LAB01-1"=w4702, "SET LAB01-1"=w4701, "TDMS LAB01-1"=w4704) -> (w4691:T32)  [unwired: 1 in]
                    n2478 = call "sub vi - cycle&temp fail v7.vi"("Amps Lo?"=w4703, "Input Cluster"=w4691, "SELECT"=w4700, "Amps Hi?"=w4699, "Result In"=w4694) -> ("(FAIL) out"=w4696:cluster{"FAIL LO":dbl, "FAIL HI":dbl}, "(DISP) out"=w4692:T4, "T-RISE"=w4693:cluster{"T-RISE (L)":dbl, "T-RISE (N)":dbl}, "Result Out"=w4695:bool, "file error"=w4698:errorcluster)  [unwired: 10 in]
                    n2479 = local write "TEMP RISE LAB01-1"(w4693) -> ()
                    n2480 = local write "FAIL LAB01-1"(w4696) -> ()
                    n2481 = local write "DISP LAB01-1"(w4692) -> ()
                    n2482 = local write "RESULT LAB01-1"(w4695) -> ()
                    n2483 = local write "data file error"(w4698) -> ()
                  }
                }
              }
              frame #1 {
                # "LAB01-2"
                n2484 = case shown="True" w4708 {
                  tunnel: w4710 -> [_ w4723]
                  tunnel: w4707 -> [_ w4720]
                  tunnel: w4709 -> [_ w4719]
                  frame False {
                  }
                  frame True {
                    n2485 = local read "TEMP START LAB01-2"() -> (w4725:cluster{"TL":dbl, "TN":dbl})
                    n2486 = local read "FAIL LAB01-2"() -> (w4716:cluster{"LO":dbl, "HI":dbl})
                    n2487 = local read "TDMS LAB01-2"() -> (w4724:refnum<k34>)
                    n2488 = local read "SET LAB01-2"() -> (w4721:T5)
                    n2489 = local read "DISP LAB01-2"() -> (w4722:T4)
                    n2490 = local read "RESULT LAB01-2"() -> (w4713:bool)
                    n2491 = local read "SIG LAB01-2"() -> (w4726:T2)
                    n2492 = Bundle("FAIL LAB01-2"=w4716, "SIG LAB01-2"=w4726, "TEMP START LAB01-2"=w4725, "DISP LAB01-2"=w4722, "SET LAB01-2"=w4721, "TDMS LAB01-2"=w4724) -> (w4711:T33)  [unwired: 1 in]
                    n2493 = call "sub vi - cycle&temp fail v7.vi"("Amps Lo?"=w4723, "Input Cluster"=w4711, "SELECT"=w4720, "Amps Hi?"=w4719, "Result In"=w4713) -> ("(FAIL) out"=w4715:cluster{"FAIL LO":dbl, "FAIL HI":dbl}, "(DISP) out"=w4718:T4, "T-RISE"=w4712:cluster{"T-RISE (L)":dbl, "T-RISE (N)":dbl}, "Result Out"=w4714:bool, "file error"=w4717:errorcluster)  [unwired: 10 in]
                    n2494 = local write "TEMP RISE LAB01-2"(w4712) -> ()
                    n2495 = local write "FAIL LAB01-2"(w4715) -> ()
                    n2496 = local write "DISP LAB01-2"(w4718) -> ()
                    n2497 = local write "RESULT LAB01-2"(w4714) -> ()
                    n2498 = local write "data file error"(w4717) -> ()
                  }
                }
              }
              frame #2 {
                # "LAB02-1"
                n2499 = case shown="True" w4728 {
                  tunnel: w4730 -> [_ w4743]
                  tunnel: w4727 -> [_ w4740]
                  tunnel: w4729 -> [_ w4739]
                  frame False {
                  }
                  frame True {
                    n2500 = local read "TEMP START LAB02-1"() -> (w4745:cluster{"TL":dbl, "TN":dbl})
                    n2501 = local read "FAIL LAB02-1"() -> (w4736:cluster{"LO":dbl, "HI":dbl})
                    n2502 = local read "TDMS LAB02-1"() -> (w4744:refnum<k34>)
                    n2503 = local read "SET LAB02-1"() -> (w4741:T5)
                    n2504 = local read "DISP LAB02-1"() -> (w4742:T4)
                    n2505 = local read "SIG LAB02-1"() -> (w4746:T2)
                    n2506 = local read "RESULT LAB02-1"() -> (w4733:bool)
                    n2507 = Bundle("FAIL LAB02-1"=w4736, "SIG LAB02-1"=w4746, "TEMP START LAB02-1"=w4745, "DISP LAB02-1"=w4742, "SET LAB02-1"=w4741, "TDMS LAB02-1"=w4744) -> (w4731:T34)  [unwired: 1 in]
                    n2508 = call "sub vi - cycle&temp fail v7.vi"("Amps Lo?"=w4743, "Input Cluster"=w4731, "SELECT"=w4740, "Amps Hi?"=w4739, "Result In"=w4733) -> ("(FAIL) out"=w4735:cluster{"FAIL LO":dbl, "FAIL HI":dbl}, "(DISP) out"=w4738:T4, "T-RISE"=w4732:cluster{"T-RISE (L)":dbl, "T-RISE (N)":dbl}, "Result Out"=w4734:bool, "file error"=w4737:errorcluster)  [unwired: 10 in]
                    n2509 = local write "TEMP RISE LAB02-1"(w4732) -> ()
                    n2510 = local write "FAIL LAB02-1"(w4735) -> ()
                    n2511 = local write "DISP LAB02-1"(w4738) -> ()
                    n2512 = local write "RESULT LAB02-1"(w4734) -> ()
                    n2513 = local write "data file error"(w4737) -> ()
                  }
                }
              }
              frame #3 {
                # "LAB02-2"
                n2514 = case shown="True" w4748 {
                  tunnel: w4750 -> [_ w4763]
                  tunnel: w4747 -> [_ w4760]
                  tunnel: w4749 -> [_ w4759]
                  frame False {
                  }
                  frame True {
                    n2515 = local read "TEMP START LAB02-2"() -> (w4765:cluster{"TL":dbl, "TN":dbl})
                    n2516 = local read "FAIL LAB02-2"() -> (w4756:cluster{"LO":dbl, "HI":dbl})
                    n2517 = local read "TDMS LAB02-2"() -> (w4764:refnum<k34>)
                    n2518 = local read "SET LAB02-2"() -> (w4761:T5)
                    n2519 = local read "DISP LAB02-2"() -> (w4762:T4)
                    n2520 = local read "SIG LAB02-2"() -> (w4766:T2)
                    n2521 = local read "RESULT LAB02-2"() -> (w4753:bool)
